vi "Dance.vi"(10 "Map":i32[](array[numeric]), 11 "Line Dancer in":refnum<class "Line Dancer.lvclass">) -> (1 "index of element":i32, 2 "Action":T1, 3 "Line Dancer out":refnum<class "Line Dancer.lvclass">)   [LabVIEW 2015, in "Line Dancer.lvclass"]
uses:
  Line Dancer.lvclass
  Type Defs/Action Enum.ctl
  Type Defs/Direction Enum.ctl
  Line Dancer Type.ctl
  Line Dancer.lvclass/Line Dancer.ctl
  Type Defs/SB Type Defs.lvlib
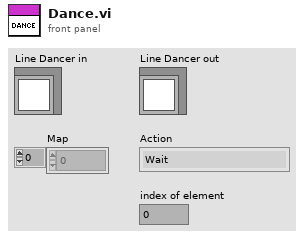
[diagram p1: front panel]
types:
  T1 = typedef "SB Type Defs.lvlib/Action Enum.ctl" = enum16{"Wait", "Move", "Attack", "Replicate"}
  T2 = typedef "SB Type Defs.lvlib/Direction Enum.ctl" = enum16{"NW", "N", "NE", "E", "SE", "S", "SW", "W"}
  T3 = typedef "Line Dancer.lvclass/Line Dancer Type.ctl" = enum16{"Top", "Bottom", "Start"}
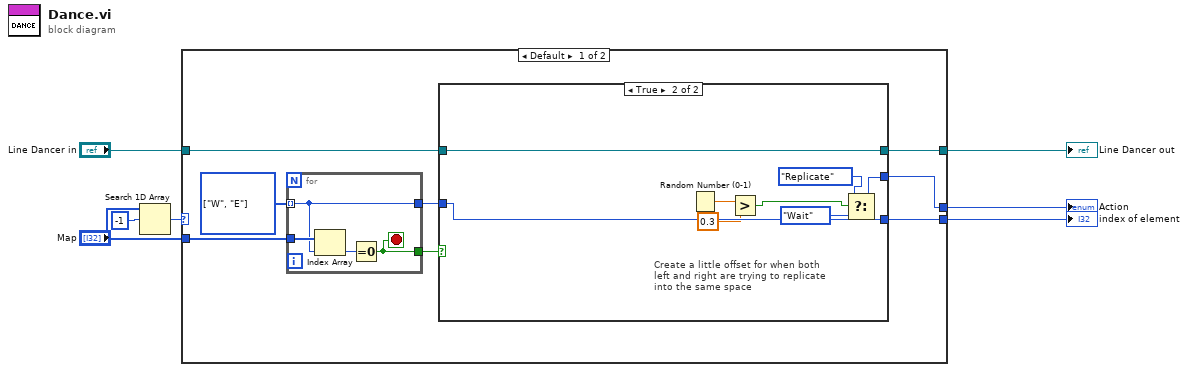
[diagram p0: block diagram]
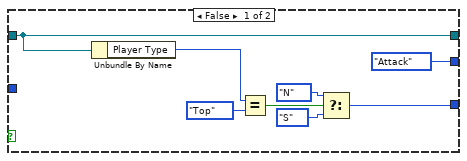
[diagram p2: hidden frame]
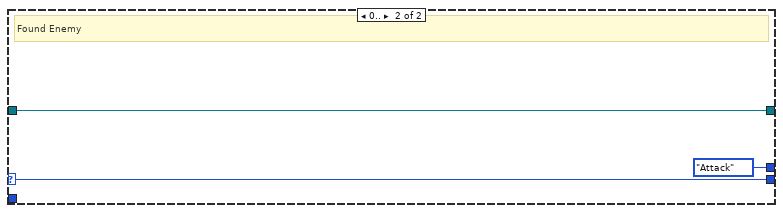
[diagram p3: hidden frame]
diagram:
  n1 = Search 1D Array(1D array="Map", element=-1) -> (index of element=w2:i32)  [unwired: 1 in]
  n2 = case shown="Default" w2 {
    selector: w2 -> [_ w37]
    tunnel: [w12 Action_Enum."Attack" ("Action")] -> w3
    tunnel: [w10 w37] -> w4
    tunnel: "Map" -> [w15 _]
    tunnel: [w8 w36] -> w7
    tunnel: "Line Dancer in" -> [w9 w36]
    frame Default {
      w14 = T2[] [enum."W", enum."E"] items=["NW", "N", "NE", "E", "SE", "S", "SW", "W"]
      n3 = for {
        tunnel: w15 -> [w35]
        tunnel: w14 -> [w34] mode=indexing
        tunnel: [w34] -> w11
        tunnel: [w32] -> w13
        stop <- w32 stop-if-true
        n4 = Index Array(array=w35, index=w34) -> (element=w33:i32)
        n5 = Equal To 0?(x=w33) -> (x = 0?=w32:bool)
      }
      n6 = case shown="True" w13 {
        tunnel: [Action_Enum."Attack" ("Action") w28] -> w12
        tunnel: [w18 w31] -> w10
        tunnel: w11 -> [_ w31]
        tunnel: w9 -> [w22 w30]
        tunnel: [w22 w30] -> w8
        frame False {
          n7 = Unbundle By Name(w22) -> ("Player Type"=w21:T3)
          n8 = Equal?(x=w21, y=Line_Dancer_Type."Top") -> (x = y?=w19:bool)
          n9 = Select(t=Direction_Enum."N" ("Direction"), s=w19, f=Direction_Enum."S" ("Direction")) -> (s? t:f=w18:T2)
        }
        frame True {
          # "Create a little offset for when both\nleft and right are trying to replicate\ninto the same space"
          n10 = Random Number (0-1)() -> (number: 0 to 1=w26:dbl)
          n11 = Greater?(x=w26, y=0.3) -> (0:w24:bool)
          n12 = Select(t=Action_Enum."Replicate" ("f"), s=w24, f=Action_Enum."Wait") -> (s? t:f=w28:T1)
        }
      }
    }
    frame 0.. {
      # "Found Enemy"
    }
  }
  "Line Dancer out" <- w7
  "index of element" <- w4
  "Action" <- w3
